vi "DAC Init Results.vi"(8 "error in":errorcluster, 9 "Log Details?":bool, 10 "tdms file":refnum<k34>, 11 "DAC Vacum Pressure in":refnum<class "DAC Vacum Pressure.lvclass">) -> (0 "error out":errorcluster, 2 "tdms file out":refnum<k34>)   [LabVIEW 2019, in "DAC.lvlib" / "DAC Vacum Pressure.lvclass"]
uses:
  DAC Vacum Pressure.lvclass
  C:/Users/krio/Documents/LV_Projects/test-stand/App/DAC/DAC.lvclass
  DAC.lvclass/DAC.ctl
  DAC Vacum Pressure.lvclass/DAC Vacum Pressure.ctl
  DAC.lvclass
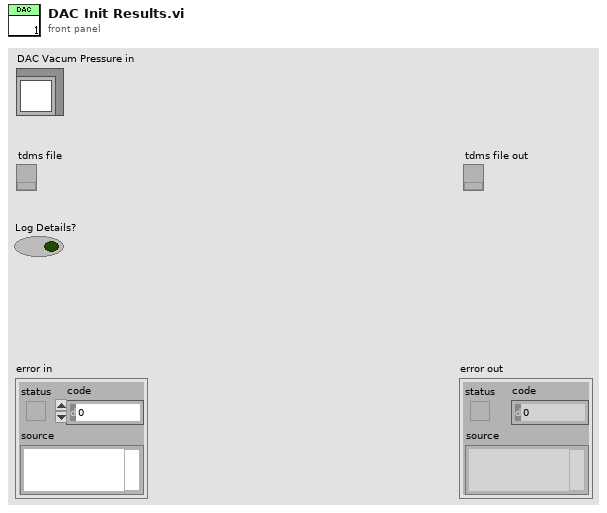
[diagram p1: front panel]
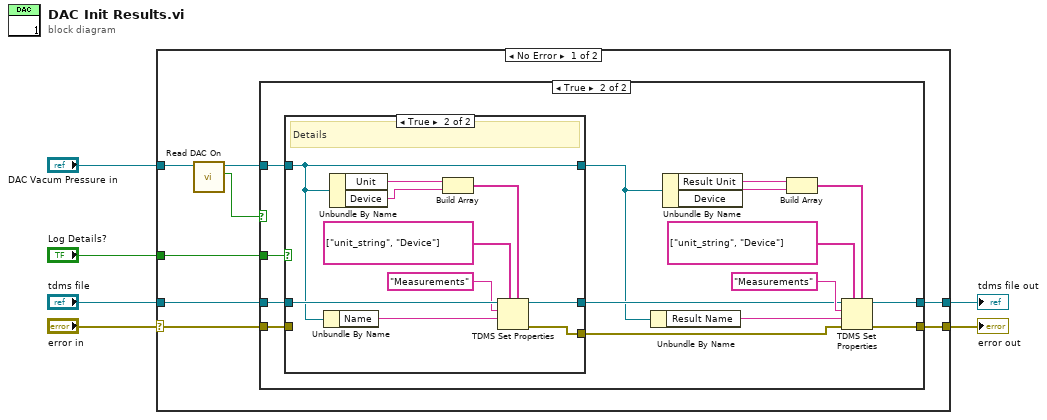
[diagram p0: block diagram]
diagram:
  n1 = case shown="No Error" "error in" {
    selector: "error in" -> [w10 w46]
    tunnel: [w7 w46] -> w6
    tunnel: "DAC Vacum Pressure in" -> [w14 _]
    tunnel: "tdms file" -> [w11 w45]
    tunnel: [w8 w45] -> w5
    tunnel: "Log Details?" -> [w9 _]
    frame No Error {
      n2 = call "Read DAC On.vi"("DAC in"=w14) -> ("DAC On"=w12:bool, "DAC out"=w13:refnum<class "DAC Vacum Pressure.lvclass">)  [unwired: 8 in, 1 out]
      n3 = case shown="True" w12 {
        tunnel: w11 -> [w15 w31]
        tunnel: [w15 w18] -> w8
        tunnel: [w16 w19] -> w7
        tunnel: w13 -> [_ w30]
        tunnel: w10 -> [w16 w17]
        tunnel: w9 -> [_ w29]
        frame False {
        }
        frame True {
          n4 = case shown="True" w29 {
            tunnel: w31 -> [w33 w44]
            tunnel: [w33 w39] -> w22
            tunnel: [w32 w38] -> w20
            tunnel: w30 -> [w34 w35]
            tunnel: [w34 w35] -> w21
            tunnel: w17 -> [w32 _]
            frame False {
            }
            frame True {
              # "Details"
              n5 = Unbundle By Name(w35) -> ("Name"=w37:string)
              n6 = Unbundle By Name(w35) -> ("Unit"=w41:string, "Device"=w36:string)
              n7 = Build Array(w41, w36) -> (w40:string[])
              n8 = TDMS Set Properties(5:w40, 7:string[] ["unit_string", "Device"] ("property names"), 9:w37, 10:"Measurements" ("group name in (Untitled)"), 11:w44) -> (0:w38:errorcluster, 3:w39:refnum<k34>)  [unwired: 1 in, 2 out]
            }
          }
          n9 = Unbundle By Name(w21) -> ("Result Name"=w24:string)
          n10 = Unbundle By Name(w21) -> ("Result Unit"=w26:string, "Device"=w23:string)
          n11 = Build Array(w26, w23) -> (w25:string[])
          n12 = TDMS Set Properties(5:w25, 7:string[] ["unit_string", "Device"] ("property names"), 8:w20, 9:w24, 10:"Measurements" ("group name in (Untitled)"), 11:w22) -> (0:w19:errorcluster, 3:w18:refnum<k34>)  [unwired: 2 out]
        }
      }
    }
    frame Error {
    }
  }
  "error out" <- w6
  "tdms file out" <- w5
